vi "update safety interlock state.vi"(7 "queues":T1, 10 "messageHandler in":T2 {"params"."controlChannels"."ballControl" items=["Module6/output0", "Module6/output1", "Module6/output2", "Module6/output3", "Not-Used"]; "params"."controlChannels"."butterflyControl" items=["Module6/output0", "Module6/output1", "Module6/output2", "Module6/output3", "Not-Used"]; "params"."controlChannels"."speedControl" items=["Module6/output0", "Module6/output1", "Module6/output2", "Module6/output3", "Not-Used"]}, 11 "vars.Interlocks":T3) -> (3 "messageHandler out":T2 {"params"."controlChannels"."ballControl" items=["Module6/output0", "Module6/output1", "Module6/output2", "Module6/output3", "Not-Used"]; "params"."controlChannels"."butterflyControl" items=["Module6/output0", "Module6/output1", "Module6/output2", "Module6/output3", "Not-Used"]; "params"."controlChannels"."speedControl" items=["Module6/output0", "Module6/output1", "Module6/output2", "Module6/output3", "Not-Used"]})   [LabVIEW 2018]
uses:
  type defs/message handler data.ctl
  customVI/liveData/state.ctl
  type defs/Queues.ctl
  <vilib>/Utility/error.llb/Error Cluster From Error Code.vi
  supporting VIs/polymorphic VIs/enqueue for message handler.vi
  supporting VIs/polymorphic VIs/enqueue for user interface.vi
  <vilib>/ErrorRing/Error Ring.xnode
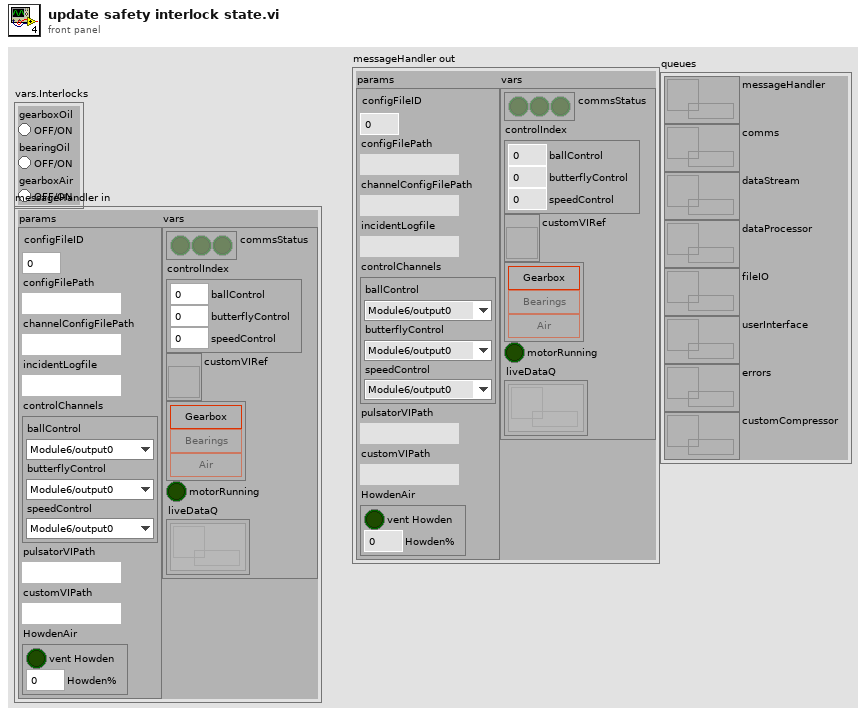
[diagram p1: front panel]
types:
  T1 = typedef "Queues.ctl" = cluster{"messageHandler":refnum<queue>, "comms":refnum<queue>, "dataStream":refnum<queue>, "dataProcessor":refnum<queue>, "fileIO":refnum<queue>, "userInterface":refnum<queue>, "errors":refnum<queue>, "customCompressor":refnum<queue>}
  T2 = typedef "message handler data.ctl" = cluster{"params":cluster{"configFileID":u32, "configFilePath":path, "channelConfigFilePath":path, "incidentLogfile":path, "controlChannels":cluster{"ballControl":u16, "butterflyControl":u16, "speedControl":u16}, "pulsatorVIPath":path, "customVIPath":path, "HowdenAir":cluster{"vent Howden":bool, "Howden%":dbl}}, "vars":cluster{"commsStatus":bool[], "controlIndex":cluster{"ballControl":u16, "butterflyControl":u16, "speedControl":u16}, "customVIRef":refnum<vi>, "Interlocks":cluster{"gearboxOil":bool, "bearingOil":bool, "gearboxAir":bool}, "motorRunning":bool, "liveDataQ":refnum<queue>[]}}
  T3 = cluster{"gearboxOil":bool, "bearingOil":bool, "gearboxAir":bool}
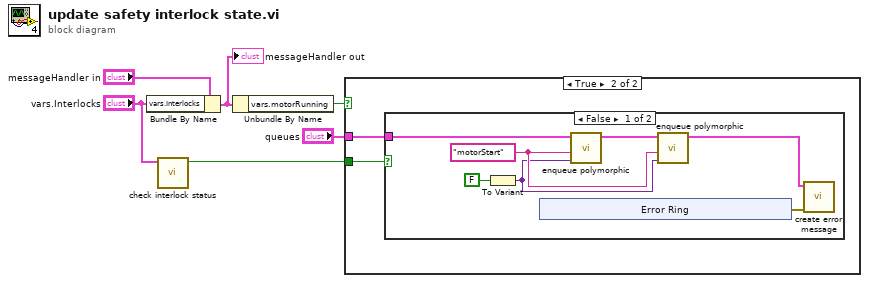
[diagram p0: block diagram]
diagram:
  n1 = Bundle By Name(cluster="messageHandler in", "vars.Interlocks"="vars.Interlocks") -> (w5:T2)
  "messageHandler out" <- w5
  n2 = call "check interlock status.vi"("Interlocks"="vars.Interlocks") -> ("interlocksOK"=w2:bool)  [unwired: 10 in]
  n3 = Unbundle By Name(w5) -> ("vars.motorRunning"=w3:bool)
  n4 = case shown="True" w3 {
    tunnel: w2 -> [_ w8]
    tunnel: "queues" -> [_ w7]
    frame False {
    }
    frame True {
      n5 = case shown="False" w8 {
        tunnel: w7 -> [w15 _]
        frame False {
          w12 = "motorStart" ("message")
          n6 = To Variant(anything=FALSE) -> (Variant=w11:variant)
          n7 = xnode "Error Ring"() -> ("error out"=w9:errorcluster)
          n8 = call-poly "enqueue polymorphic.vi"("data"=w11, "message"=w12, "Queues"=w15) -> ("Queues out"=w13:T1)  [unwired: 8 in]
          n9 = call-poly "enqueue polymorphic.vi"("data"=w11, "message"=w12, "Queues"=w13) -> ("Queues out"=w10:T1)  [unwired: 8 in]
          n10 = call "create error message.vi"("error in (no error)"=w9, "queues"=w10) -> ()  [unwired: 10 in]
        }
        frame True {
        }
      }
    }
  }
